vi "GenerateCode.vi"(0 "XRef":T15, 1 "Terms":T12, 2 "Diagram":T11, 3 "State In":T1 {"BlockNodeState"."Draw Style" items=["FunctionBlock", "ExpressVI", "Variable", "Elemental I/O", "32x32 Icon", "FunctionBlockCompact"]; "BlockNodeState"."Terminal Data"."Terminal Flags" format="%.0b"}) -> (14 "Generated Code?":T10, 15 "Reply":T8, 16 "State Out":T1 {"BlockNodeState"."Draw Style" items=["FunctionBlock", "ExpressVI", "Variable", "Elemental I/O", "32x32 Icon", "FunctionBlockCompact"]; "BlockNodeState"."Terminal Data"."Terminal Flags" format="%.0b"})   [LabVIEW 2020, in "NI_ExpressFull.lvlib" / "ExpressSpectralMeasurementsBlockNode.xnode"]
uses:
  <vilib>/express/express analysis/Spectral/XNode/ExpressSpectralMeasurementsBlockNode.xnode
  <vilib>/XNodeSupport/NI_XNodeSupport.lvlib
  <vilib>/Utility/traverseref.llb/TRef TravTarget.ctl
  <vilib>/XNodeSupport/XNodeXNodeRef.ctl
  <vilib>/XNodeSupport/XNodeTermRef.ctl
  <vilib>/XNodeSupport/XNodeTermIDPair.ctl
  <vilib>/XNodeSupport/XNodeTermIDPairs.ctl
  <vilib>/XNodeSupport/XNodeTopLevelDiagramRef.ctl
  <vilib>/XNodeSupport/XNodeBool.ctl
  <vilib>/XNodeSupport/XNodeStringArray.ctl
  <vilib>/XNodeSupport/XNodeString.ctl
  <vilib>/picture/picture.llb/imagedata.ctl
  <vilib>/BlockNodeSupport/BlockNodeState.ctl
  <vilib>/express/express analysis/Spectral/XNode/State.ctl
  <vilib>/express/express shared/XNodes/controls/ExpressState.ctl
  <vilib>/BlockNodeSupport/TerminalData.ctl
  <vilib>/XNodeSupport/XNodeType.ctl
  <vilib>/express/express shared/XNodes/controls/ExpressTerminalInfo.ctl
panel:
  in  "Path":path
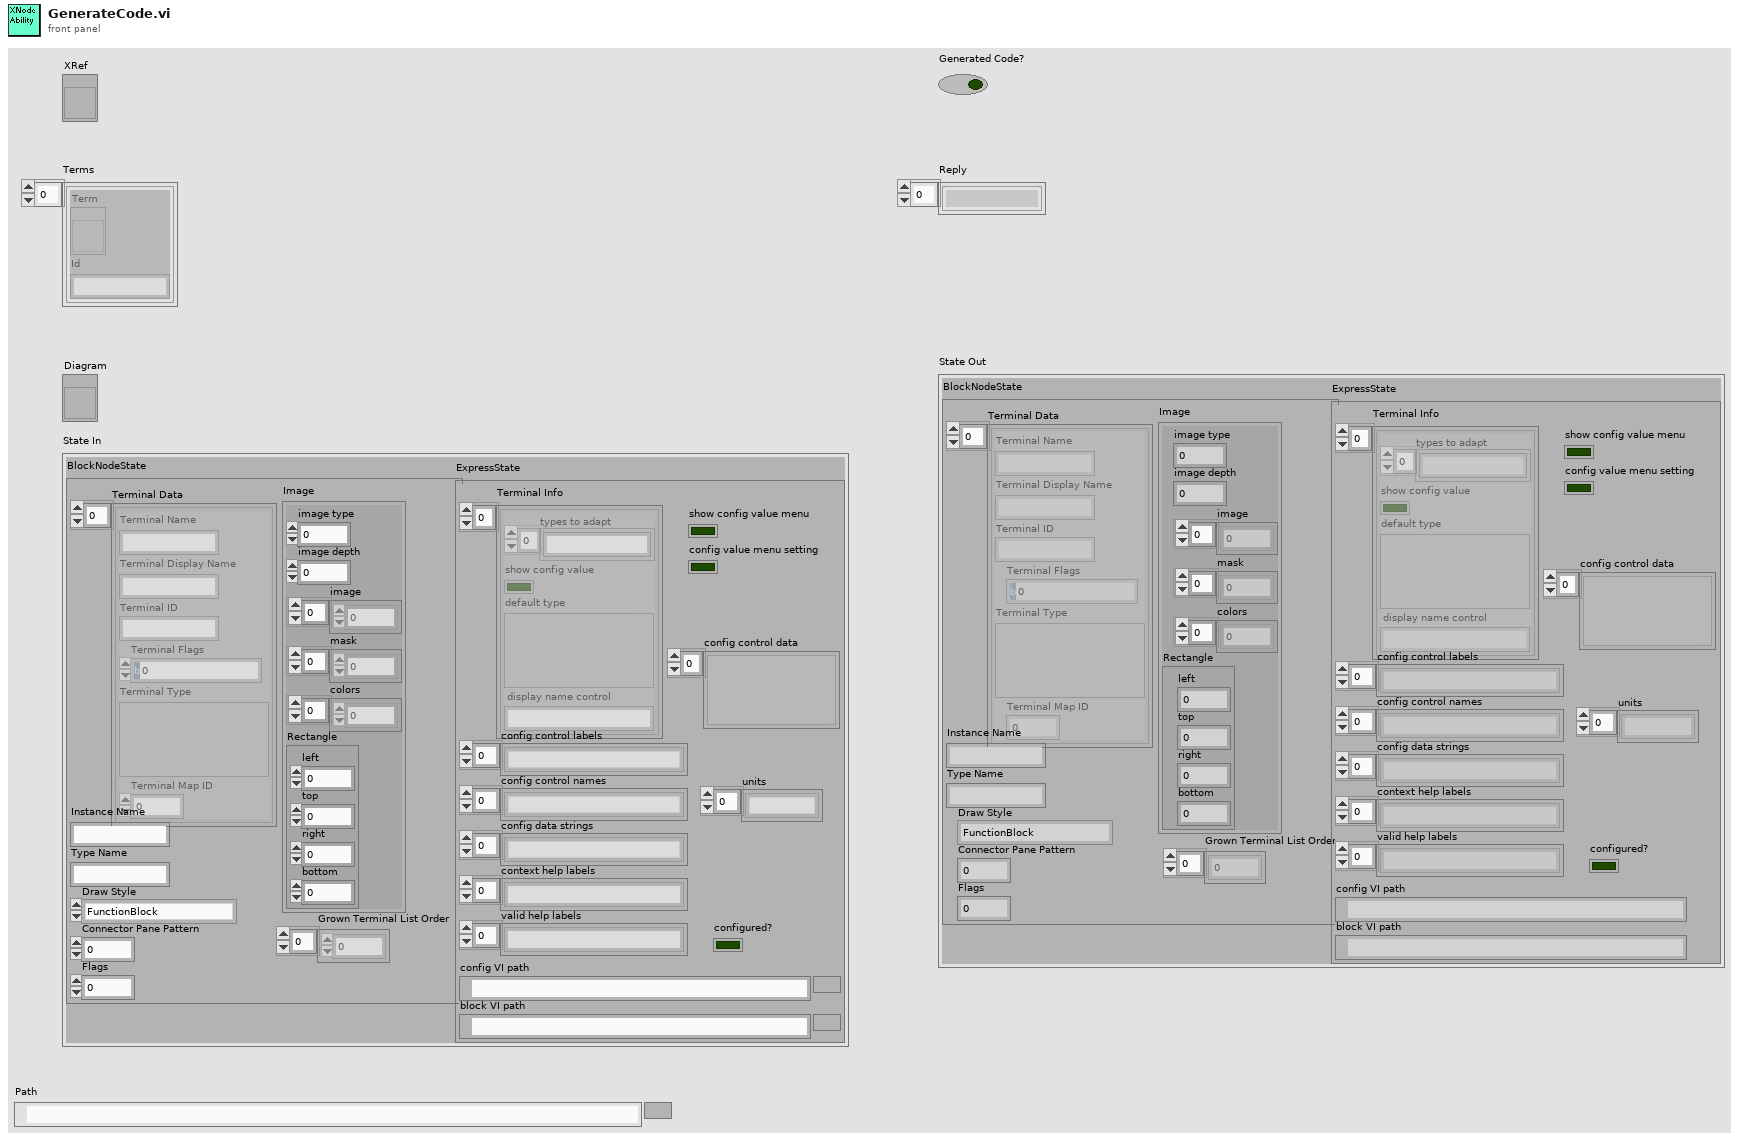
[diagram p1: front panel]
types:
  T1 = typedef "NI_ExpressFull.lvlib/ExpressSpectralMeasurementsBlockNode.xnode/State.ctl" = cluster{"BlockNodeState":T2, "ExpressState":T5}
  T2 = typedef "BlockNodeState.ctl" = cluster{"Terminal Data":T3[], "Instance Name":string, "Type Name":string, "Draw Style":i32, "Connector Pane Pattern":i32, "Flags":i32, "Grown Terminal List Order":i32[], "Image":T4}
  T3 = typedef "TerminalData.ctl" = cluster{"Terminal Name":string, "Terminal Display Name":string, "Terminal ID":string, "Terminal Flags":i32, "Terminal Type":variant, "Terminal Map ID":i32}
  T4 = typedef "imagedata.ctl" = cluster{"image type":i32, "image depth":i32, "image":u8[], "mask":u8[], "colors":u32[], "Rectangle":cluster{"left":i16, "top":i16, "right":i16, "bottom":i16}}
  T5 = typedef "ExpressState.ctl" = cluster{"Terminal Info":T6, "config control names":string[], "config data strings":string[], "config control data":variant[], "units":string[], "configured?":bool, "config VI path":path, "block VI path":path, "config control labels":string[], "show config value menu":bool, "config value menu setting":bool, "context help labels":string[], "valid help labels":string[]}
  T6 = typedef "ExpressTerminalInfo.ctl" = cluster{"types to adapt":string[], "show config value":bool, "default type":T7, "display name control":string}[]
  T7 = typedef "NI_XNodeSupport.lvlib/XNodeType.ctl" = variant
  T8 = typedef "NI_XNodeSupport.lvlib/XNodeStringArray.ctl" = T9[]
  T9 = typedef "NI_XNodeSupport.lvlib/XNodeString.ctl" = string
  T10 = typedef "NI_XNodeSupport.lvlib/XNodeBool.ctl" = bool
  T11 = typedef "NI_XNodeSupport.lvlib/XNodeTopLevelDiagramRef.ctl" = refnum<vi>
  T12 = typedef "NI_XNodeSupport.lvlib/XNodeTermIDPairs.ctl" = T13[]
  T13 = typedef "NI_XNodeSupport.lvlib/XNodeTermIDPair.ctl" = cluster{"Term":T14, "Id":T9}
  T14 = typedef "NI_XNodeSupport.lvlib/XNodeTermRef.ctl" = refnum<vi>
  T15 = typedef "NI_XNodeSupport.lvlib/XNodeXNodeRef.ctl" = refnum<vi>
  T16 = enum32{"Magnitude (RMS)", "Magnitude (Peak)", "Power spectrum", "Power spectral density"}
  T17 = typedef "TRef TravTarget.ctl" = enum16{"FP", "BD", "Other"}
  T18 = enum32{"None", "Size to Fit", "Arrange Horizontally", "Arrange Vertically"}
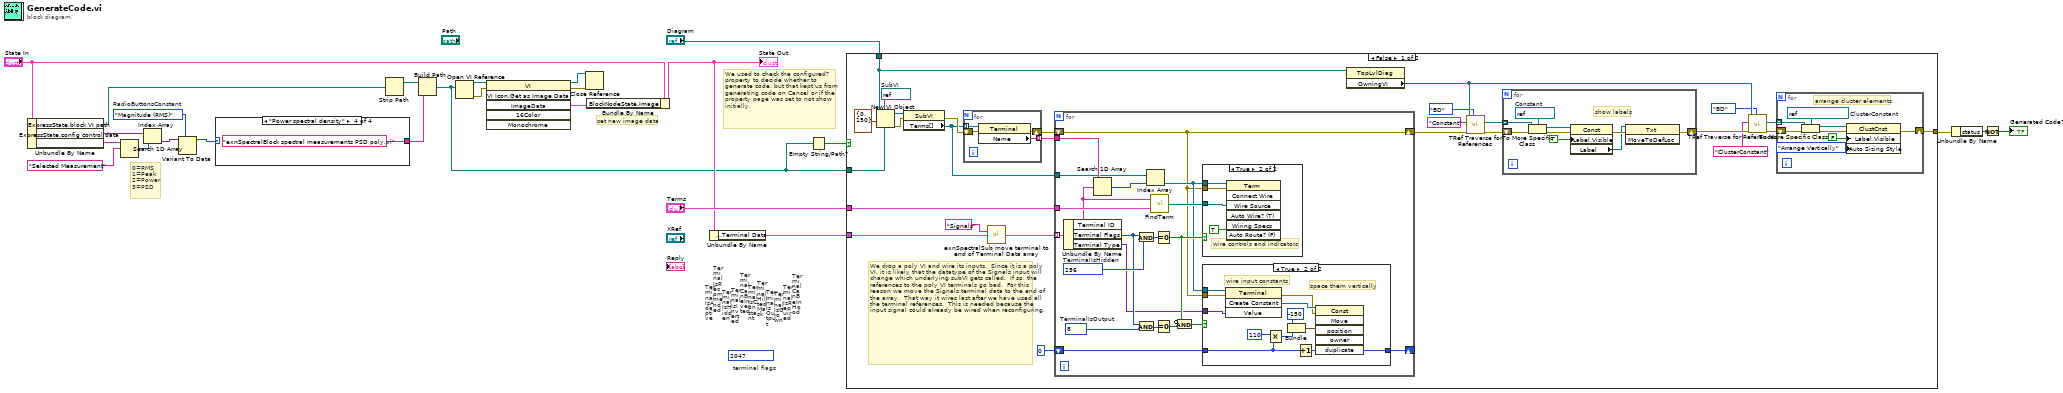
[diagram p0: block diagram]
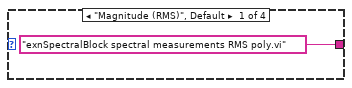
[diagram p2: hidden frame]
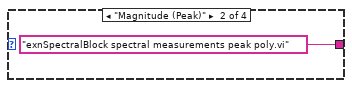
[diagram p3: hidden frame]
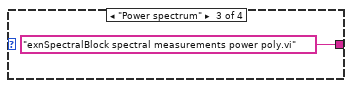
[diagram p4: hidden frame]
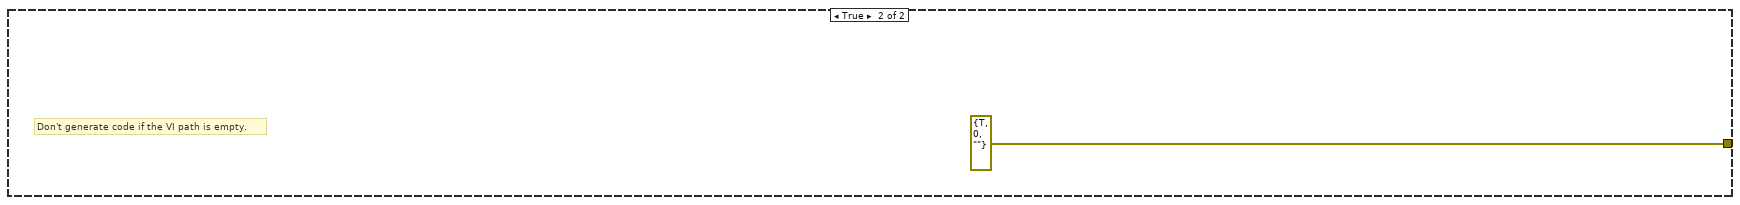
[diagram p7: hidden frame]
diagram:
  w4 = T16."Magnitude (RMS)"  # RadioButtonsConstant
  (unwired) 2047 ("TermFlags")
  # "We used to check the configured? property to decide whether to generate code, but that kept us from generating code on Cancel or if the property page was set to not show initially."
  # "TerminalIsAdaptive"
  # "TerminalIsRecommended"
  # "TerminalIsHidden"
  # "terminal flags"
  # "TerminalIsInverted"
  # "TerminalCanBeInverted"
  # "TerminalIsConstant"
  # "TerminalHilitedMask"
  # "TerminalIsOutput"
  # "TerminalIsGrown"
  # "TerminalIsRequired"
  # "TerminalCanBeInHood"
  # "0=RMS\n1=Peak\n2=Power\n3=PSD"
  # "set new image data"
  n1 = Unbundle By Name("State In") -> ("ExpressState.block VI path"=w11:path, "ExpressState.config control data"=w15:variant[], "ExpressState.config control labels"=w13:string[])
  n2 = Search 1D Array(1D array=w13, element="Selected Measurement" ("y")) -> (index of element=w14:i32)  [unwired: 1 out]
  n3 = Index Array(array=w15, index=w14) -> (element=w3:variant)
  n4 = Variant To Data(type=w4, Variant=w3) -> (data=w2:T16)  [unwired: 1 in, 1 out]
  n5 = case shown="\"Power spectral density\"" w2 {
    tunnel: ["exnSpectralBlock spectral measurements RMS poly.vi" ("y") "exnSpectralBlock spectral measurements peak poly.vi" ("y") "exnSpectralBlock spectral measurements power poly.vi" ("y") "exnSpectralBlock spectral measurements PSD poly.vi" ("y")] -> w9
    frame "Magnitude (RMS)", Default {
    }
    frame "Magnitude (Peak)" {
    }
    frame "Power spectrum" {
    }
    frame "Power spectral density" {
    }
  }
  n6 = Strip Path(path=w11) -> (stripped path=w8:path)  [unwired: 1 out]
  n7 = Build Path(base path=w8, name or relative path=w9) -> (appended path=w10:path)
  n8 = Open VI Reference(vi path=w10) -> (vi reference=w18:refnum<vi>, error out=w5:errorcluster)  [unwired: 1 in, 4 out]
  n9 = invoke class="VI" method="VI Icon.Get as Image Data"(reference=w18, error in=w5) -> (reference out=w6:refnum<vi>, error out=w7:errorcluster, "ImageData"=w17:T4)  [unwired: 4 in, 3 out]
  n10 = Close Reference(reference=w6, error in (no error)=w7) -> ()  [unwired: 1 out]
  n11 = Bundle By Name(cluster="State In", "BlockNodeState.Image"=w17) -> (w19:T1)
  "State Out" <- w19
  n12 = Unbundle By Name(w19) -> ("BlockNodeState.Terminal Data"=w22:T3[])
  n13 = Empty String/Path?(string/path=w10) -> (empty?=w1:bool)
  n14 = case shown="False" w1 {
    tunnel: [w40 errorcluster {"status"=TRUE, "code"=0, "source"=""} ("error out")] -> w21
    tunnel: w10 -> [w47 _]
    tunnel: "Diagram" -> [w42 _]
    tunnel: "Terms" -> [w48 _]
    tunnel: w22 -> [w46 _]
    frame False {
      w56 = refnum<vi> refnum  # SubVI
      # "We drop a poly VI and wire its inputs.  Since it is a poly VI, it is likely that the datatype of the Signals input will change which underlying subVI gets called.  If so, the references to the poly VI terminals go bad.  For this reason we move the Signals terminal data to the end of the array.  That way it wires last after we have used all the terminal references.  This is needed because the input signal could already be wired when reconfiguring."
      n15 = New VI Object(vi object class=w56, owner refnum=w42, position/next to=cluster{"Horizontal":i16, "Vertical":i16} {"Horizontal"=0, "Vertical"=150}, 6:w47) -> (object refnum=w49:refnum<vi>, 0:w54:errorcluster)  [unwired: 1 in, 3 out]
      n16 = property class="SubVI"(reference=w49, error in=w54) -> (error out=w53:errorcluster, "Terms[]"=w50:refnum<vi>[])  [unwired: 1 out]
      n17 = for {
        tunnel: w50 -> [w110] mode=indexing
        shift-right: [w112] -> w52
        shift-left: w53 -> [w113]
        tunnel: [w111] -> w51 mode=indexing
        n18 = property class="Terminal"(reference=w110, error in=w113) -> (error out=w112:errorcluster, "Name"=w111:string)  [unwired: 1 out]
      }
      n19 = call <vilib>:"exnSpectralSub move terminal to end of Terminal Data array.vi"("Terminal ID"="Signals", "Terminal Data in"=w46) -> ("Terminal Data out"=w45:T3[])  [unwired: 13 out]
      n20 = for {
        tunnel: w45 -> [w93] mode=indexing
        tunnel: w51 -> [w92]
        tunnel: w50 -> [w91]
        shift-right: [w78] -> w30
        shift-left: w52 -> [w78]
        tunnel: w48 -> [w89]
        shift-right: [w75] -> _
        shift-left: 0 ("Left") -> [w76]
        w86 = 8  # TerminalIsOutput
        w88 = 256  # TerminalIsHidden
        n21 = Unbundle By Name(w93) -> ("Terminal ID"=w74:string, "Terminal Flags"=w85:i32, "Terminal Type"=w80:variant)
        n22 = Search 1D Array(1D array=w92, element=w74) -> (index of element=w90:i32)  [unwired: 1 out]
        n23 = And(x=w85, y=w88) -> (x .and. y?=w87:i32)
        n24 = And(x=w85, y=w86) -> (x .and. y?=w84:i32)
        n25 = Index Array(array=w91, index=w90) -> (element=w79:refnum<vi>)
        n26 = call <vilib>:"FindTerm.vi"("Terms"=w89, "String"=w74) -> ("Term"=w81:refnum<vi>)
        n27 = Equal To 0?(x=w87) -> (x = 0?=w83:bool)
        n28 = Equal To 0?(x=w84) -> (x = 0?=w82:bool)
        n29 = Compound Arithmetic op=AND(invert w83, w82) -> (w77:bool)
        n30 = case shown="True" w83 {
          tunnel: w79 -> [_ w109]
          tunnel: w78 -> [_ w108]
          tunnel: w81 -> [_ w107]
          frame False {
            # "hidden - don't wire"
          }
          frame True {
            # "wire controls and indicators"
            n31 = invoke class="Term" method="Connect Wire"(reference=w109, error in=w108, "Wire Source"=w107, "Auto Route? (F)"=TRUE) -> ()  [unwired: 3 in, 7 out]
          }
        }
        n32 = case shown="True" w77 {
          tunnel: w79 -> [_ w105]
          tunnel: w80 -> [_ w104]
          tunnel: w78 -> [_ w103]
          tunnel: w76 -> [w94 w97]
          tunnel: [w94 w96] -> w75
          frame False {
          }
          frame True {
            # "space them vertically"
            # "wire input constants"
            n33 = invoke class="Terminal" method="Create Constant"(reference=w105, error in=w103, "Value"=w104) -> (error out=w95:errorcluster, "Create Constant"=w102:refnum<vi>)  [unwired: 1 in, 2 out]
            n34 = Multiply(x=110 ("Left"), y=w97) -> (x*y=w99:i32)
            n35 = Bundle("Left"=-150, w99) -> (w100:cluster{"Left":i32, i32})  [unwired: 1 out]
            n36 = Increment(x=w97) -> (x+1=w96:i32)
            n37 = invoke class="Const" method="Move"(reference=w102, error in=w95, "position"=w100) -> ()  [unwired: 3 in, 6 out]
          }
        }
      }
      n38 = property class="TopLvlDiag"(reference=w42) -> ("OwningVI"=w41:refnum<vi>)  [unwired: 1 in, 2 out]
      n39 = call <vilib>:"TRef Traverse for References.vi"("Traverse Target"=TRef_TravTarget."BD", "error in (no error)"=w30, "Class Name"="Constant", "VI Refnum"=w41) -> ("error out"=w37:errorcluster, "References"=w36:refnum<vi>[])  [unwired: 1 in, 5 out]
      n40 = for {
        tunnel: w36 -> [w65] mode=indexing
        shift-right: [w67] -> w35
        shift-left: w37 -> [w73]
        w72 = refnum<vi> refnum  # Constant
        # "show labels"
        n41 = To More Specific Class(target class=w72, reference=w65, error in=w73) -> (specific class reference=w69:refnum<vi>, error out=w70:errorcluster)
        n42 = property class="Const"(reference=w69, error in=w70, "Label.Visible"=TRUE) -> (error out=w68:errorcluster, "Label"=w66:refnum<vi>)  [unwired: 1 out]
        n43 = invoke class="Txt" method="MoveToDefLoc"(reference=w66, error in=w68) -> (error out=w67:errorcluster)  [unwired: 1 in, 2 out]
      }
      n44 = call <vilib>:"TRef Traverse for References.vi"("Traverse Target"=TRef_TravTarget."BD", "error in (no error)"=w35, "Class Name"="ClusterConstant", "VI Refnum"=w41) -> ("error out"=w33:errorcluster, "References"=w34:refnum<vi>[])  [unwired: 1 in, 5 out]
      n45 = for {
        tunnel: w34 -> [w60] mode=indexing
        shift-right: [w57] -> w40
        shift-left: w33 -> [w64]
        w63 = refnum<vi> refnum  # ClusterConstant
        # "arrange cluster elements"
        n46 = To More Specific Class(target class=w63, reference=w60, error in=w64) -> (specific class reference=w61:refnum<vi>, error out=w62:errorcluster)
        n47 = property class="ClustCnst"(reference=w61, error in=w62, "Label.Visible"=FALSE, "Auto Sizing Style"=T18."Arrange Vertically") -> (error out=w57:errorcluster)  [unwired: 1 out]
      }
    }
    frame True {
      # "Don't generate code if the VI path is empty."
    }
  }
  n48 = Unbundle By Name(w21) -> ("status"=w25:bool)
  n49 = Not(x=w25) -> (.not. x?=→"Generated Code?":bool)
